vi "Andor_iXon_Cooling.vi"(8 "Boolean array in":bool[](array[boolean]), 10 "target temperature / [°C]":i32, 11 "Cooling":bool) -> (0 "Boolean array out":bool[](array[boolean]))   [LabVIEW 2009]
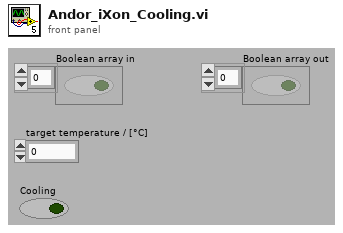
[diagram p1: front panel]
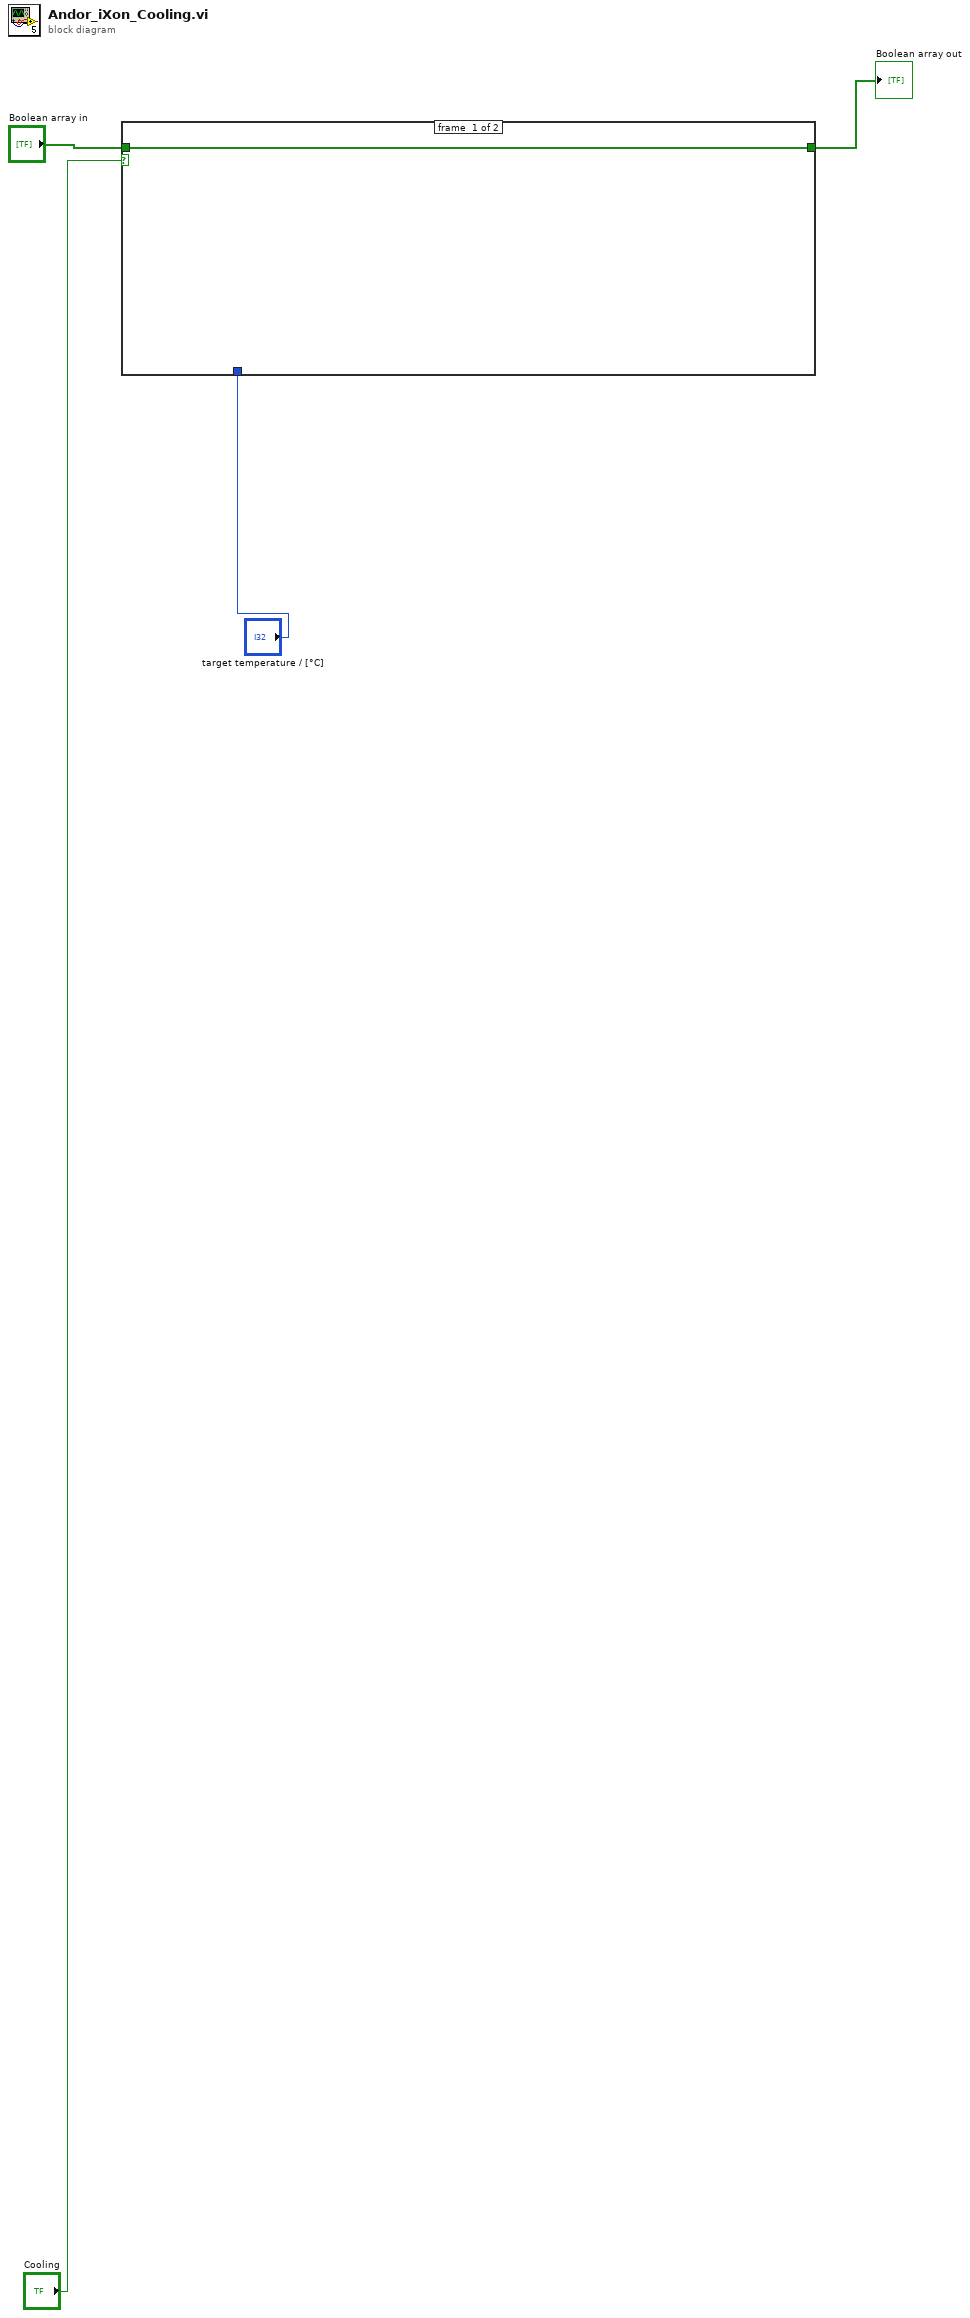
[diagram p0: block diagram]
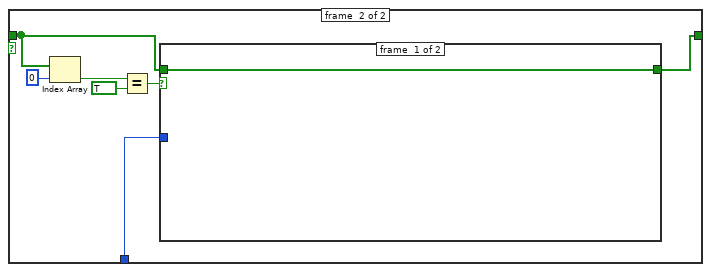
[diagram p2: hidden frame]
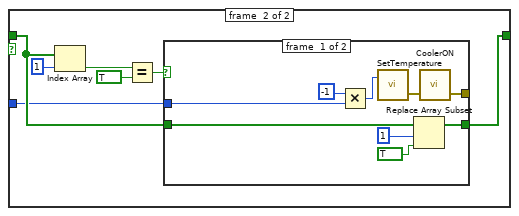
[diagram p3: hidden frame]
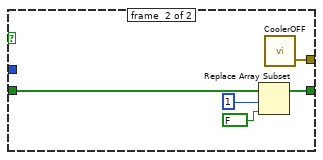
[diagram p4: hidden frame]
diagram:
  n1 = case shown="True" "Cooling" {
    tunnel: "Boolean array in" -> [w5 w8]
    tunnel: [w5 w7] -> w2
    tunnel: "target temperature / [°C]" -> [_ w6]
    frame #0 {
    }
    frame #1 {
      n2 = Index Array(array=w8, index=0) -> (element=w11:bool)
      n3 = Equal?(x=w11, y=TRUE) -> (x = y?=w9:bool)
      n4 = case shown="True" w9 {
        tunnel: w8 -> [w13 w16]
        tunnel: [w13 w15] -> w7
        tunnel: w6 -> [_ w14]
        frame #0 {
        }
        frame #1 {
          n5 = Index Array(array=w16, index=1) -> (element=w19:bool)
          n6 = Equal?(x=w19, y=TRUE) -> (x = y?=w17:bool)
          n7 = case shown="False" w17 {
            tunnel: w16 -> [w27 w34]
            tunnel: [w26 w32] -> w15
            tunnel: [w25 w31] -> _
            tunnel: w14 -> [w21 _]
            frame #0 {
              n8 = Multiply(x=-1, y=w21) -> (x*y=w23:i32)
              n9 = call "SetTemperature.vi"("temperature"=w23) -> ("error out"=w22:errorcluster)  [unwired: 1 in, 1 out]
              n10 = Replace Array Subset(array=w27, new element=TRUE, index=1) -> (w26:bool[])
              n11 = call "CoolerON.vi"("error in (no error)"=w22) -> ("error out"=w25:errorcluster)  [unwired: 2 out]
            }
            frame #1 {
              n12 = Replace Array Subset(array=w34, new element=FALSE, index=1) -> (w32:bool[])
              n13 = call "CoolerOFF.vi"() -> ("error out"=w31:errorcluster)  [unwired: 1 in, 2 out]
            }
          }
        }
      }
    }
  }
  "Boolean array out" <- w2
